vi "Send AT Command.vi"(9 "AT Command":string, 11 "UDP Output Port":refnum<k16>) -> (3 "UDP Output Port":refnum<k16>)   [LabVIEW 2011]
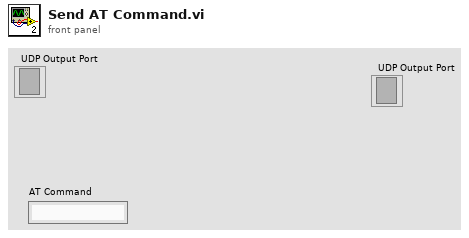
[diagram p1: front panel]
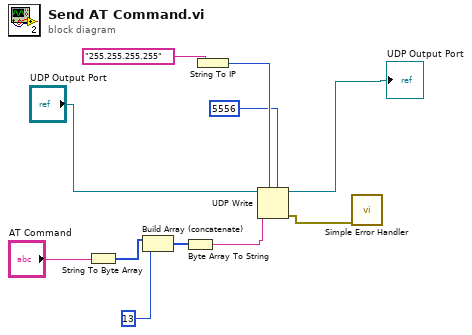
[diagram p0: block diagram]
diagram:
  n1 = String To Byte Array(string="AT Command") -> (unsigned byte array=w4:u8[])
  n2 = Build Array (concatenate)(w4, u8 13) -> (w5:u8[])
  n3 = Byte Array To String(unsigned byte array=w5) -> (string=w2:string)
  n4 = String To IP(1:"255.255.255.255") -> (0:w10:u32)
  n5 = UDP Write(address=w10, port or service name=u16 5556, connection ID="UDP Output Port", data in=w2) -> (error out=w6:errorcluster, 3:→"UDP Output Port":refnum<k16>)  [unwired: 2 in]
  n6 = call <vilib>:"Simple Error Handler.vi"("error in (no error)"=w6) -> ()  [unwired: 4 in, 5 out]
